vi "GB_Local Sense Test_v2.vi"(7 "error in (no error)":errorcluster, 9 "HMP VISA":refnum<visa-resource-name>, 10 "Control Board VISA":refnum<visa-resource-name>) -> (0 "error out":errorcluster, 2 "Voltage Readings":dbl[][](array[numeric]), 3 "Pass?":bool)   [LabVIEW 2022 SP3]
uses:
  HMP4000 Communication/HMP4040_ChannelControlAutomatic.ctl
panel:
  out "MSE Array":dbl[](array[numeric])
  out "Message OUT":string
  in  "Message IN":string
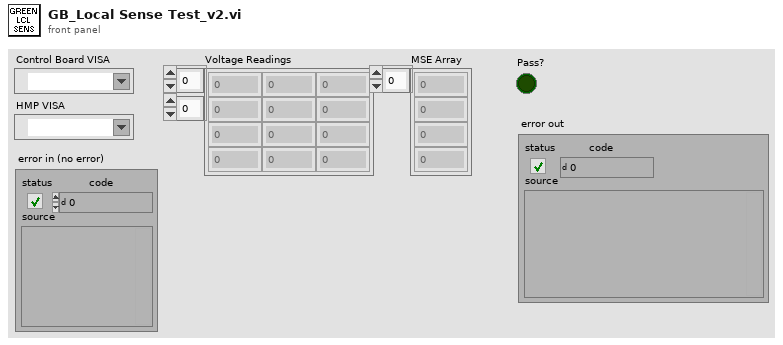
[diagram p1: front panel]
types:
  T1 = typedef "HMP4040_ChannelControlAutomatic.ctl" = enum16{"Off", "Control Power", "HMP2020 Control + DC32V", "HMP2020 Control + DC8V", "HMP4040 Control + DC32V", "HMP4040 Control +DC8V", "HMP4040 Ch2 24V 4A"}
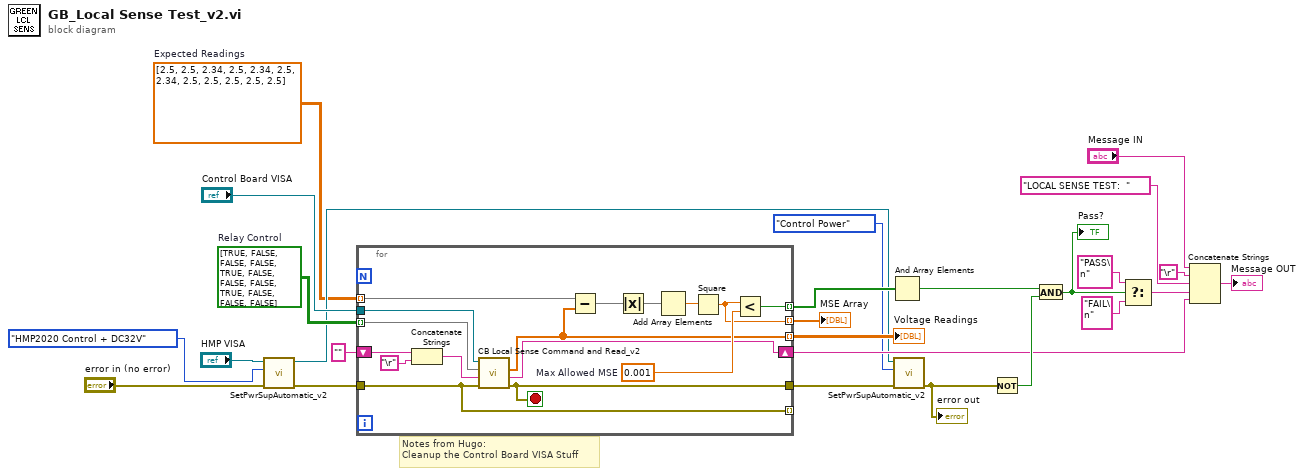
[diagram p0: block diagram]
diagram:
  w1 = dbl[][] [[2.5, 2.5, 2.34], [2.5, 2.34, 2.5], [2.34, 2.5, 2.5], [2.5, 2.5, 2.5]]  # Expected Readings
  w25 = bool[][] [[TRUE, FALSE, FALSE], [FALSE, TRUE, FALSE], [FALSE, FALSE, TRUE], [FALSE, FALSE, FALSE]]  # Relay Control
  # "Notes from Hugo:\nCleanup the Control Board VISA Stuff"
  n1 = call "SetPwrSupAutomatic_v2.vi"("error in (no error)"="error in (no error)", "Enum"=HMP4040_ChannelControlAutomatic."HMP2020 Control + DC32V", "HMP VISA"="HMP VISA") -> ("error out"=w8:errorcluster, "HMP VISA Out"=w5:refnum<visa-resource-name>)  [unwired: 7 in]
  n2 = for {
    tunnel: [w42] -> w7
    tunnel: [w27] -> _ mode=indexing
    tunnel: w1 -> [w39] mode=indexing
    tunnel: [w36] -> w26 mode=indexing
    tunnel: w25 -> [w35] mode=indexing
    tunnel: [w34] -> w22 mode=indexing
    tunnel: [w33] -> w21 mode=indexing
    shift-right: [w32] -> w14
    shift-left: "" -> [w31]
    tunnel: "Control Board VISA" -> [w28]
    tunnel: w8 -> [w27]
    stop <- w42 stop-if-true
    w37 = 0.001  # Max Allowed MSE
    n3 = Concatenate Strings(w31, "\r") -> (w30:string)
    n4 = call "CB Local Sense Command and Read_v2.vi"("error in (no error)"=w27, "Message IN"=w30, "Relay Control"=w35, "Control Board VISA"=w28) -> ("error out"=w42:errorcluster, "Message OUT"=w32:string, "Voltage Array"=w34:dbl[])  [unwired: 4 in, 1 out]
    n5 = Subtract(x=w39, y=w34) -> (x-y=w41:dbl[])
    n6 = Absolute Value(x=w41) -> (abs(x)=w40:dbl[])
    n7 = Add Array Elements(numeric array=w40) -> (sum=w38:dbl)
    n8 = Square(x=w38) -> (x^2=w33:dbl)
    n9 = Less?(x=w33, y=w37) -> (x < y?=w36:bool)
  }
  "Voltage Readings" <- w22
  "MSE Array" <- w21
  n10 = And Array Elements(Boolean array=w26) -> (logical AND=w24:bool)
  n11 = call "SetPwrSupAutomatic_v2.vi"("error in (no error)"=w7, "Enum"=HMP4040_ChannelControlAutomatic."Control Power", "HMP VISA"=w5) -> ("error out"=w6:errorcluster)  [unwired: 7 in, 1 out]
  "error out" <- w6
  n12 = Not(x=w6) -> (.not. x?=w23:bool)
  n13 = And(x=w24, y=w23) -> (x .and. y?=w16:bool)
  "Pass?" <- w16
  n14 = Select(t="PASS\n", s=w16, f="FAIL\n") -> (s? t:f=w15:string)
  n15 = Concatenate Strings("Message IN", "\r", "LOCAL SENSE TEST:  ", w15, w14) -> (→"Message OUT":string)
